vi "Initialize.vi"(8 "error in (no error)":errorcluster, 10 "Major Frame":refnum<class "Major Frame.lvclass">, 11 "Configuration":T1) -> (0 "error out":errorcluster, 3 "Bus Controller out":refnum<class "Bus Controller.lvclass">)   [LabVIEW 2020, in "BCI-1553 API.lvlib" / "Bus Controller.lvclass"]
doc: "Generates a Bus Controller subcomponent object. There can only be a single Bus Controller (and nothing else) present in a Component. The Bus Controller must be initialized with a Major Frame that is already setup with a valid schedule, Messages, and Minor Frames."
uses:
  Bus Controller.lvclass
  TypeDefs/Bus Controller Configuration.ctl
  TypeDefs/Bus Controller Timeout.ctl
  Frames & Messages/Major Frame/Major Frame.lvclass
  Bus Controller.lvclass/Bus Controller.ctl
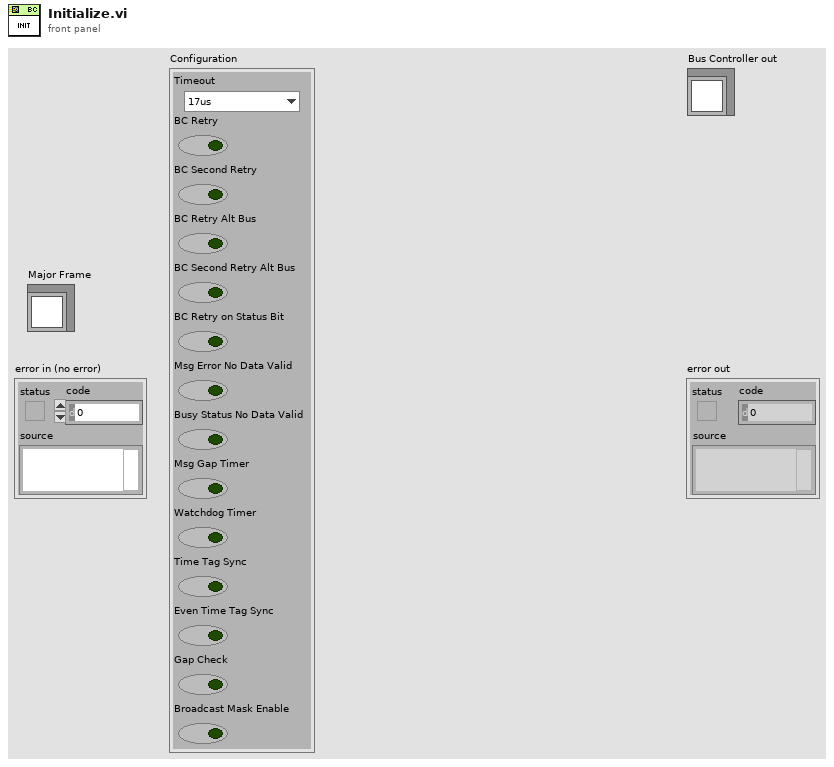
[diagram p1: front panel]
types:
  T1 = typedef "BCI-1553 API.lvlib/Bus Controller.lvclass/Bus Controller Configuration.ctl" = cluster{"Timeout":T2, "BC Retry":bool, "BC Second Retry":bool, "BC Retry Alt Bus":bool, "BC Second Retry Alt Bus":bool, "BC Retry on Status Bit":bool, "Msg Error No Data Valid":bool, "Busy Status No Data Valid":bool, "Msg Gap Timer":bool, "Watchdog Timer":bool, "Time Tag Sync":bool, "Even Time Tag Sync":bool, "Gap Check":bool, "Broadcast Mask Enable":bool}
  T2 = typedef "BCI-1553 API.lvlib/Bus Controller.lvclass/Bus Controller Timeout.ctl" = enum16{"17us", "22us", "60us", "140us"}
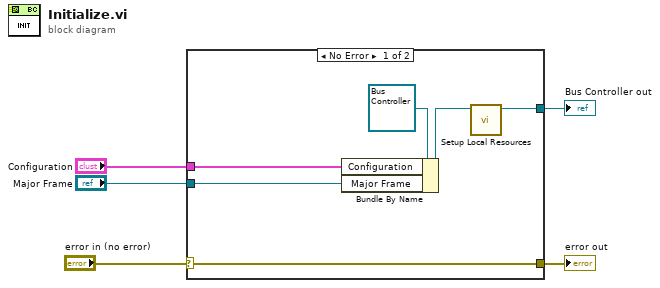
[diagram p0: block diagram]
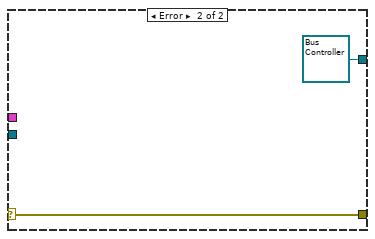
[diagram p2: hidden frame]
diagram:
  n1 = case shown="No Error" "error in (no error)" {
    selector: "error in (no error)" -> [w11 w13]
    tunnel: [w11 w13] -> w4
    tunnel: [w7 refnum<class "Bus Controller.lvclass"> refnum ("Bus Controller out")] -> w3
    tunnel: "Configuration" -> [w9 _]
    tunnel: "Major Frame" -> [w6 _]
    frame No Error {
      n2 = Bundle By Name(cluster=refnum<class "Bus Controller.lvclass"> refnum ("Bus Controller out"), "Configuration"=w9, "Major Frame"=w6) -> (w8:refnum<class "Bus Controller.lvclass">)
      n3 = call-dynamic "Setup Local Resources.vi"("1553 SubComponent in"=w8) -> ("1553 SubComponent out"=w7:refnum<class "Bus Controller.lvclass">)  [unwired: 9 in, 1 out]
    }
    frame Error {
    }
  }
  "error out" <- w4
  "Bus Controller out" <- w3
